vi "Create Queue.vi"(8 "error in (no error)":errorcluster, 11 "name (unnamed)":string) -> (0 "error out":errorcluster, 3 "Message Queue Out":refnum<queue>)   [LabVIEW 2020]
uses:
  Controls/QMH Message Cluster.ctl
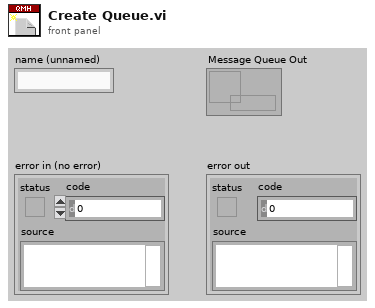
[diagram p1: front panel]
types:
  T1 = typedef "QMH Message Cluster.ctl" = cluster{"Message":string, "Data":variant}
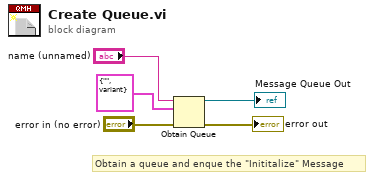
[diagram p0: block diagram]
diagram:
  # "Obtain a queue and enque the \"Inititalize\" Message"
  n1 = Obtain Queue(name (unnamed)="name (unnamed)", element data type=T1 {"Message"="", "Data"=variant} ("QMH Message"), error in (no error)="error in (no error)") -> (queue out=→"Message Queue Out":refnum<queue>, error out=→"error out":errorcluster)  [unwired: 2 in, 1 out]
